vi "EdgeDetection.vi"() -> ()   [LabVIEW 2016]
uses:
  <vilib>/vision/NI_Vision_Development_Module.lvlib
panel:
  in  "File Path":path
  out "Line Profile":cluster{"x0":sgl, "dx":sgl, "Pixels Line":sgl[]}(graph)
  in  "Process":u16(ring) items=["Get First Edge", "Get First + Last Edge", "Get All Edges", "Get Best Edge"]
  in  "Edge Options":T1={"Edge Polarity"=2, "Kernel Size"=37, "Width"=5, "Minimum Edge Strength"=10.0, "Interpolation Type"=0, "Data Processing Method"=1} {"Edge Polarity" items=["All Edges", "Rising Edges", "Falling Edges"]; "Interpolation Type" items=["Zero Order"=0, "Bilinear"=1, "Bilinear Fixed"=4]; "Data Processing Method" items=["Average", "Median"]}
  in  "Enum":enum16{"B2T", "L2R", "R2L", "T2B"}(ring)
  in  "Y":dbl format="%#_13g"
  in  "X":dbl format="%#_13g"
  out "Line Equation":cluster{"A":dbl, "B":dbl, "C":dbl} {"C" format="%.2f"; "B" format="%.2f"; "A" format="%.2f"}
  in  "Path":path=path "C:/Users/TTUHEP/Documents/LabVIEW/image3.png"
  out "Image":T2(plugin-control)
  # "Ax + By + C = 0"
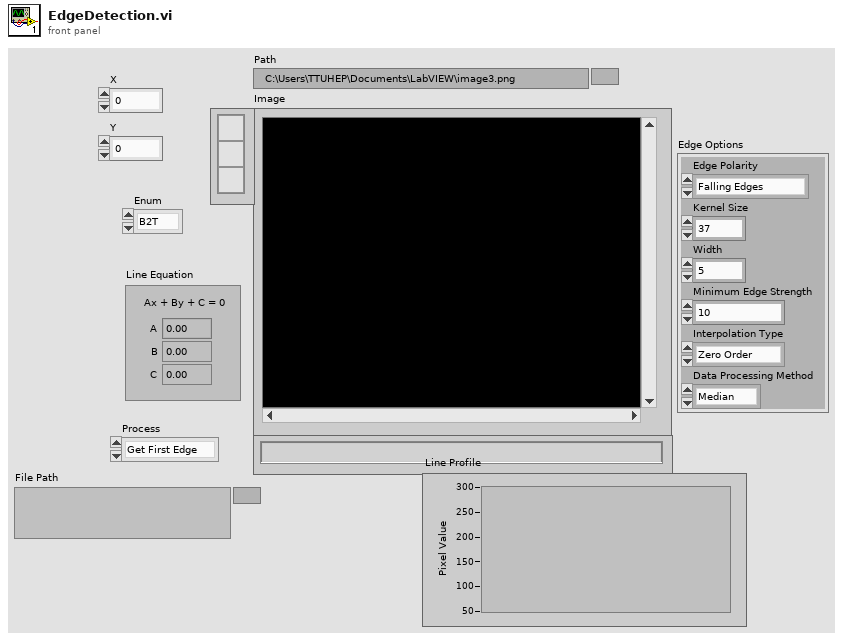
[diagram p1: front panel]
types:
  T1 = cluster{"Edge Polarity":u16, "Kernel Size":u32, "Width":u32, "Minimum Edge Strength":dbl, "Interpolation Type":u16, "Data Processing Method":u16}
  T2 = typedef "IMAQ Image.ctl" = refnum<image>
  T3 = typedef "IMAQ Line" = cluster{"Start X":i32, "Start Y":i32, "End X":i32, "End Y":i32}
  T4 = typedef "ROI Descriptor" = cluster{"Global Rectangle":i32[], "Contours":cluster{"ID":enum32{"External", "Internal"}, "Type":u32, "Coordinates":i32[]}[]}
  T5 = typedef "Edge New.ctl" = cluster{"Location (Pixel)":cluster{"X":sgl, "Y":sgl}, "Location (Real-World)":cluster{"X":sgl, "Y":sgl}, "Distance (Pixel)":dbl, "Distance (Real-World)":dbl, "Strength":dbl, "Noise":dbl, "Rising?":bool}
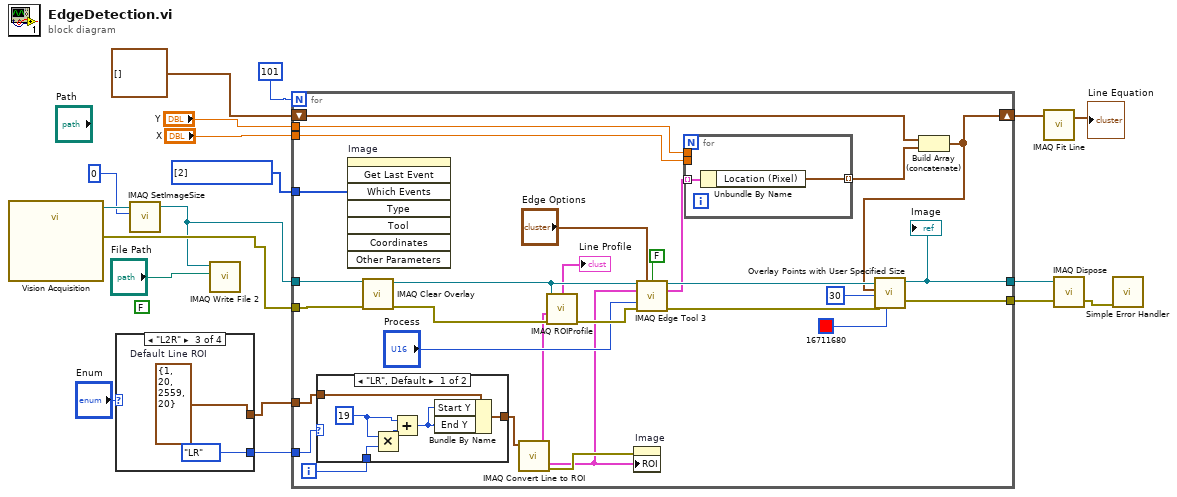
[diagram p0: block diagram]
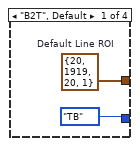
[diagram p2: hidden frame]
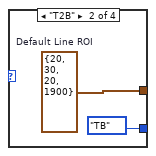
[diagram p3: hidden frame]
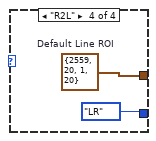
[diagram p4: hidden frame]
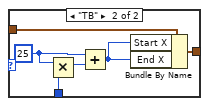
[diagram p5: hidden frame]
diagram:
  (unwired) FALSE ("Compress? (N)")
  w16 = i32[] [2] items=["No  event", "Click event", "Draw event", "Move event", "Size event", "Scroll event", "Activate event", "Close event", "Double click event"] ("Events list (all)")
  n1 = call "Vision Acquisition"() -> ("Image Out"=w3:T2, "error out"=w5:errorcluster)  [unwired: 26 in]
  n2 = case shown="\"L2R\"" "Enum" {
    tunnel: [w20 w22 w23 w25] -> w7
    tunnel: [enum16{"LR", "TB"}."TB" enum16{"LR", "TB"}."TB" enum16{"LR", "TB"}."LR" enum16{"LR", "TB"}."LR"] -> w6
    frame "B2T", Default {
      w20 = T3 {"Start X"=20, "Start Y"=1919, "End X"=20, "End Y"=1}  # Default Line ROI
    }
    frame "T2B" {
      w22 = T3 {"Start X"=20, "Start Y"=30, "End X"=20, "End Y"=1900}  # Default Line ROI
    }
    frame "L2R" {
      w23 = T3 {"Start X"=1, "Start Y"=20, "End X"=2559, "End Y"=20}  # Default Line ROI
    }
    frame "R2L" {
      w25 = T3 {"Start X"=2559, "Start Y"=20, "End X"=1, "End Y"=20}  # Default Line ROI
    }
  }
  n3 = call "IMAQ SetImageSize"("X Resolution"=0, "Image"=w3) -> ("Image Out"=w2:T2)  [unwired: 3 in, 1 out]
  n4 = call-poly "IMAQ Write File 2"("File Path"="File Path", "Image"=w2) -> ()  [unwired: 8 in, 2 out]
  n5 = for {
    N: 101 -> [_]
    tunnel: w2 -> [w52]
    tunnel: w5 -> [w51]
    shift-right: [w37] -> w12
    shift-left: cluster{"X":sgl, "Y":sgl}[] [] -> [w39]
    tunnel: w16 -> [w53]
    tunnel: [w42] -> w15
    tunnel: [w36] -> w14
    tunnel: w7 -> [w30]
    tunnel: "X" -> [w33]
    tunnel: "Y" -> [w32]
    tunnel: w6 -> [w29]
    i -> [w28]
    n6 = case shown="\"LR\", Default" w29 {
      tunnel: w28 -> [w58 w66]
      tunnel: [w60 w62] -> w31
      tunnel: w30 -> [w59 w61]
      frame "LR", Default {
        w55 = 19
        n7 = Multiply(x=w55, y=w58) -> (x*y=w56:i32)
        n8 = Add(x=w55, y=w56) -> (x+y=w57:i32)
        n9 = Bundle By Name(cluster=w59, "Start Y"=w57, "End Y"=w57) -> (w60:T3)
      }
      frame "TB" {
        w64 = 25
        n10 = Multiply(x=w64, y=w66) -> (x*y=w65:i32)
        n11 = Add(x=w64, y=w65) -> (x+y=w63:i32)
        n12 = Bundle By Name(cluster=w61, "Start X"=w63, "End X"=w63) -> (w62:T3)
      }
    }
    n13 = invoke on="Image" class="ImageControl" method="Get Last Event"("Which Events"=w53) -> ()  [unwired: 7 in, 8 out]
    n14 = call "IMAQ Clear Overlay"("error in (no error)"=w51, "Image"=w52) -> ("error out"=w50:errorcluster, "Image Out"=w49:T2)  [unwired: 8 in]
    n15 = call "IMAQ Convert Line to ROI"("Line"=w31) -> ("error out"=w54:errorcluster, "ROI Descriptor"=w34:T4)  [unwired: 8 in]
    n16 = call "IMAQ ROIProfile"("error in (no error)"=w50, "ROI Descriptor"=w34, "Image"=w49) -> ("error out"=w48:errorcluster, "ROI Graph"=→"Line Profile":cluster{"x0":sgl, "dx":sgl, "Pixels Line":sgl[]})  [unwired: 1 in, 3 out]
    n17 = property on="Image" class="ImageControl"(error in=w54, "ROI"=w34) -> ()  [unwired: 1 in, 2 out]
    n18 = call "IMAQ Edge Tool 3"("Image"=w49, "Edge Options"="Edge Options", "Optimized Mode"=FALSE, "ROI Descriptor"=w34, "Process"="Process", "error in (no error)"=w48) -> ("Image (duplicate)"=w44:T2, "Edge Information"=w40:T5[], "error out"=w43:errorcluster)  [unwired: 5 in, 2 out]
    n19 = for {
      tunnel: w40 -> [w68] mode=indexing
      tunnel: [w67] -> w38 mode=indexing
      tunnel: w33 -> [_]
      tunnel: w32 -> [_]
      n20 = Unbundle By Name(w68) -> ("Location (Pixel)"=w67:cluster{"X":sgl, "Y":sgl})
    }
    n21 = Build Array (concatenate)(w39, w38) -> (w37:cluster{"X":sgl, "Y":sgl}[])
    n22 = call "Overlay Points with User Specified Size.vi"("Color"=u32 16711680, "error in"=w43, "Point Diameter (5)"=30, "Points"=w37, "Image In"=w44) -> ("error out"=w36:errorcluster, "Image Out"=w42:T2)  [unwired: 5 in]
    "Image" <- w42
  }
  n23 = call "IMAQ Fit Line"("Points"=w12) -> ("Line Equation"=→"Line Equation":cluster{"A":dbl, "B":dbl, "C":dbl})  [unwired: 5 in, 5 out]
  n24 = call "IMAQ Dispose"("Image"=w15, "error in (no error)"=w14) -> ("error out"=w13:errorcluster)  [unwired: 4 in]
  n25 = call <vilib>:"Simple Error Handler.vi"("error in (no error)"=w13) -> ()  [unwired: 4 in, 5 out]
